vi "HOST_new.vi"() -> ()   [LabVIEW 2018]
uses:
  <instrlib>/niDMM/nidmm.llb/niDMM Function.ctl
  <instrlib>/niDMM/nidmm.llb/niDMM Resolution in Digits.ctl
  <instrlib>/niDMM/nidmm.llb/niDMM Configure Measurement Digits.vi
panel:
  out "T(t)":dbl(graph)=398.0450506439805
  out "Temp, K":dbl caption="Measurement" format="%.5f"
  out "Volts (Temp)":dbl caption="Measurement" format="%.5f"
  in  "Stop":bool
  in  "Temp Range\n(Volts)":dbl=2.0 format="%.2p"
  out "Out of Range (V, Temp)":bool caption="Signal Out of Range"
  in  "Temp":refnum<k15>="PXI1Slot6_3"
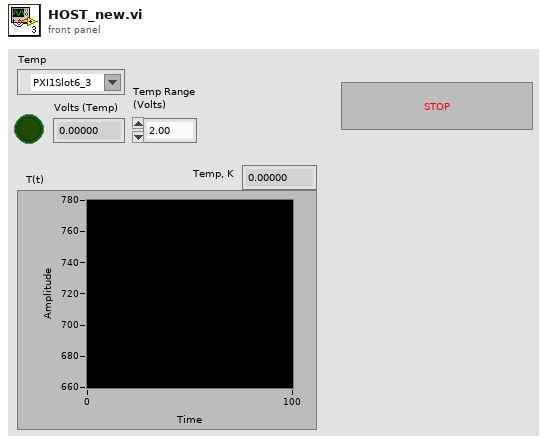
[diagram p1: front panel]
types:
  T1 = typedef "niDMM Function.ctl" = enum16{"DC Volts", "AC Volts", "DC Current", "AC Current", "2-wire Resistance", "4-wire Resistance", "Diode", "Frequency", "Period", "AC Volts DC Coupled", "Capacitance", "Inductance", "Temperature"}
  T2 = typedef "niDMM Resolution in Digits.ctl" = dbl
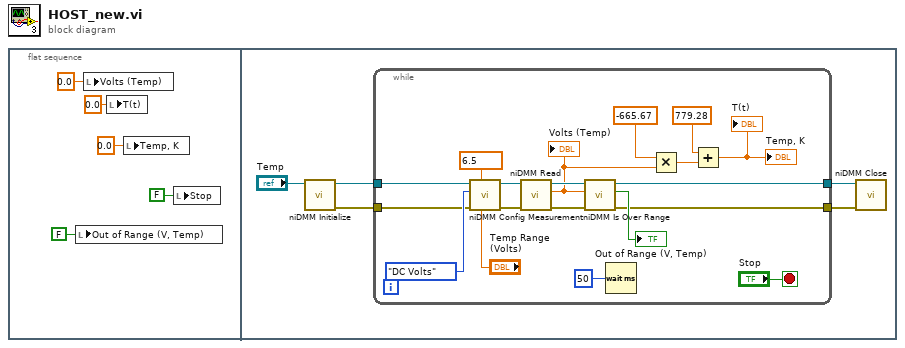
[diagram p0: block diagram]
diagram:
  n1 = flat-sequence {
    frame #0 {
      n2 = local write "Out of Range (V, Temp)"(FALSE ("Out of Range (V, Temp)")) -> ()
      n3 = local write "Volts (Temp)"(0.0 ("Volts (Temp)")) -> ()
      n4 = local write "T(t)"(0.0 ("T(t)")) -> ()
      n5 = local write "Temp, K"(0.0 ("Temp, K")) -> ()
      n6 = local write "Stop"(FALSE ("Stop")) -> ()
    }
    frame #1 {
      n7 = call <instrlib>:"niDMM Initialize.vi"("Instrument Descriptor"="Temp") -> ("error out"=w6:errorcluster, "instrument handle out"=w7:refnum<k15>)  [unwired: 9 in]
      n8 = while {
        tunnel: [w21] -> w9
        tunnel: [w20] -> w8
        tunnel: w7 -> [w18]
        tunnel: w6 -> [w17]
        stop <- "Stop" stop-if-true
        w22 = T2 6.5 items=["3 1/2"=3.5, "4 1/2"=4.5, "5 1/2"=5.5, "6 1/2"=6.5, "7 1/2"=7.5] ("Resolution in Digits")
        n9 = call-poly <instrlib>:"niDMM Config Measurement.vi"("Range"="Temp Range\n(Volts)", "Resolution in Digits"=w22, "error in (no error)"=w17, "Function"=niDMM_Function."DC Volts", "instrument handle"=w18) -> ("error out"=w28:errorcluster, "instrument handle out"=w27:refnum<k15>)  [unwired: 5 in]
        n10 = call <instrlib>:"niDMM Read.vi"("error in (no error)"=w28, "instrument handle"=w27) -> ("error out"=w25:errorcluster, "Measurement"=w16:dbl, "instrument handle out"=w24:refnum<k15>)  [unwired: 7 in]
        "Volts (Temp)" <- w16
        n11 = call <instrlib>:"niDMM Is Over Range.vi"("error in (no error)"=w25, "Measurement"=w16, "instrument handle"=w24) -> ("error out"=w20:errorcluster, "Over Range?"=→"Out of Range (V, Temp)":bool, "instrument handle out"=w21:refnum<k15>)  [unwired: 6 in]
        n12 = Wait (ms)(milliseconds to wait=u32 50) -> ()  [unwired: 1 out]
        n13 = Multiply(x=-665.67, y=w16) -> (x*y=w14:dbl)
        n14 = Add(x=779.28, y=w14) -> (x+y=→"Temp, K" →"T(t)":dbl)
      }
      n15 = call <instrlib>:"niDMM Close.vi"("error in (no error)"=w8, "instrument handle"=w9) -> ()  [unwired: 9 in, 1 out]
    }
  }
